vi "NewFile.vi"(7 "LVWS Req":refnum<class "Web Request.lvclass">) -> ()   [LabVIEW 2014]
uses:
  <vilib>/wsapi/Web Request.lvclass
  Controller/Controls/Enqueuer Enum.ctl
  File Actor/Messages/To/Change File MSG/Change File MSG.lvclass
  Controller/Controller.lvclass
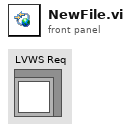
[diagram p1: front panel]
types:
  T1 = typedef "Controller.lvlib/Controller.lvclass/Enqueuer Enum.ctl" = enum8{"PAS", "CRDS", "File", "O3Lamp"}
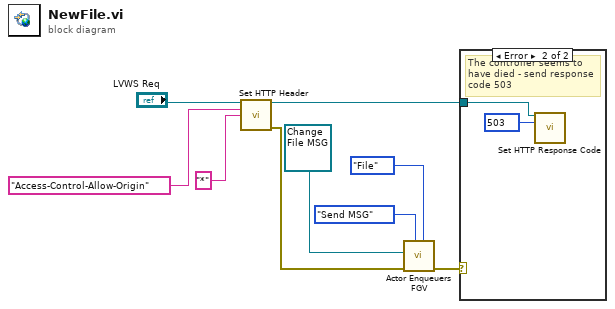
[diagram p0: block diagram]
diagram:
  n1 = call <vilib>:"Set HTTP Header.vi"("LabVIEW Web Service Request"="LVWS Req", "header"="Access-Control-Allow-Origin", "header value"="*") -> ("LabVIEW Web Service Request out"=w7:refnum<class "Web Request.lvclass">, "error out"=w2:errorcluster)  [unwired: 11 in]
  n2 = call "Actor Enqueuers FGV.vi"("Enqueuer"=Enqueuer_Enum."File", "State"=enum16{"Store", "Send MSG"}."Send MSG", "error in"=w2, "MSG"=refnum<class "Change File MSG.lvclass"> refnum ("File Library.lvlib:Change File MSG")) -> ("error out"=w1:errorcluster)  [unwired: 7 in]
  n3 = case shown="Error" w1 {
    tunnel: w7 -> [_ w10]
    frame No Error {
    }
    frame Error {
      w11 = 503 items=["100"=100, "101"=101, "200"=200, "201"=201, "202"=202, "203"=203, "204"=204, "205"=205, "206"=206, "300"=300, "301"=301, "302"=302, "303"=303, "304"=304, "305"=305, "306"=306, "307"=307, "400"=400, "401"=401, "402"=402, "403"=403, "404"=404, "405"=405, "406"=406, "407"=407, "408"=408, "409"=409, "410"=410, "411"=411, "412"=412, "413"=413, "414"=414, "415"=415, "416"=416, "417"=417, "500"=500, "501"=501, "502"=502, "503"=503, "504"=504, "505"=505] ("response code (200)")
      # "The controller seems to have died - send response code 503"
      n4 = call <vilib>:"Set HTTP Response Code.vi"("LabVIEW Web Service Request"=w10, "response code (200)"=w11) -> ()  [unwired: 12 in, 2 out]
    }
  }
